vi "Draw Scaled Image.vi"(9 "Image":T1, 10 "Picture Ref":refnum<vi>) -> ()   [LabVIEW 2020, in "VolatusGUIControls.lvlib" / "ImageButtonEditorPanel.lvclass"]
uses:
  ImageButtonEditorPanel.lvclass
  ImageButtonEditorPanel.lvclass/ImageButtonEditorPanel.ctl
  <vilib>/picture/picture.llb/imagedata.ctl
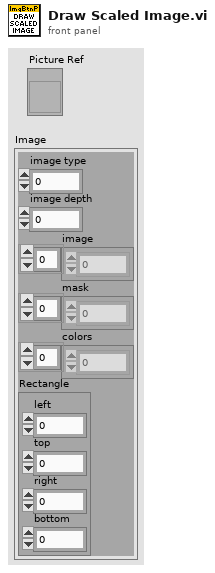
[diagram p1: front panel]
types:
  T1 = typedef "imagedata.ctl" = cluster{"image type":i32, "image depth":i32, "image":u8[], "mask":u8[], "colors":u32[], "Rectangle":cluster{"left":i16, "top":i16, "right":i16, "bottom":i16}}
  T2 = typedef "LVBoundsTypeDef.ctl" = cluster{"Width":u32, "Height":u32}
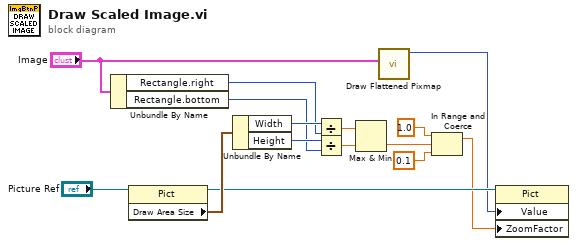
[diagram p0: block diagram]
diagram:
  n1 = Unbundle By Name("Image") -> ("Rectangle.right"=w11:i16, "Rectangle.bottom"=w12:i16)
  n2 = property class="Pict"(reference="Picture Ref") -> (reference out=w8:refnum<vi>, "Draw Area Size"=w15:T2)  [unwired: 1 in, 1 out]
  n3 = Unbundle By Name(w15) -> ("Width"=w14:u32, "Height"=w13:u32)
  n4 = Divide(x=w14, y=w11) -> (x/y=w10:dbl)
  n5 = Divide(x=w13, y=w12) -> (x/y=w9:dbl)
  n6 = Max & Min(x=w10, y=w9) -> (min(x,y)=w7:dbl)  [unwired: 1 out]
  n7 = call <vilib>:"Draw Flattened Pixmap.vi"("image data"="Image") -> ("new picture"=w4:picture)  [unwired: 8 in]
  n8 = In Range and Coerce(upper limit=1.0, x=w7, lower limit=0.1) -> (coerced(x)=w1:dbl)  [unwired: 1 out]
  n9 = property class="Pict"(reference=w8, "Value"=w4, "ZoomFactor"=w1) -> ()  [unwired: 1 in, 2 out]
